vi "MFCDialog.vi"(8 "Error In":errorcluster, 11 "MFC Configuration In":T1={"COM Port"=1, "Timeout (msec)"=100, "Setpoint"=0.0, "Valve State"=enum."Automatic", "Gas"=enum."Air", "Units"=enum."scc/m", "Serial Number"="", "Firmware Version"=""}) -> (0 "Error Out":errorcluster, 2 "Cancelled?":bool, 3 "MFC Configuration Out":T1={"COM Port"=1, "Timeout (msec)"=100, "Setpoint"=0.0, "Valve State"=enum."Automatic", "Gas"=enum."Air", "Units"=enum."scc/m", "Serial Number"="", "Firmware Version"=""})   [LabVIEW 2012]
uses:
  MFCConfiguration.ctl
  libs/Sierra-M100/Public/Controls/ValveState.ctl
  libs/Sierra-M100/Public/Controls/Gas.ctl
  libs/Sierra-M100/Public/Controls/Units.ctl
  libs/LV-Utilities/LV-Utilities.lvlib
  libs/Sierra-M100/Sierra-M100.lvlib
panel:
  in  "COM Port":u8=1
  in  "Valve State":enum16{"Automatic", "Closed", "Purge"}(ring)
  in  "Setpoint":dbl=nan format="%.1f"
  in  "CANCEL":bool
  in  "DONE":bool
  # "COM Port"
  # "Valve State"
  # "Flow Rate"
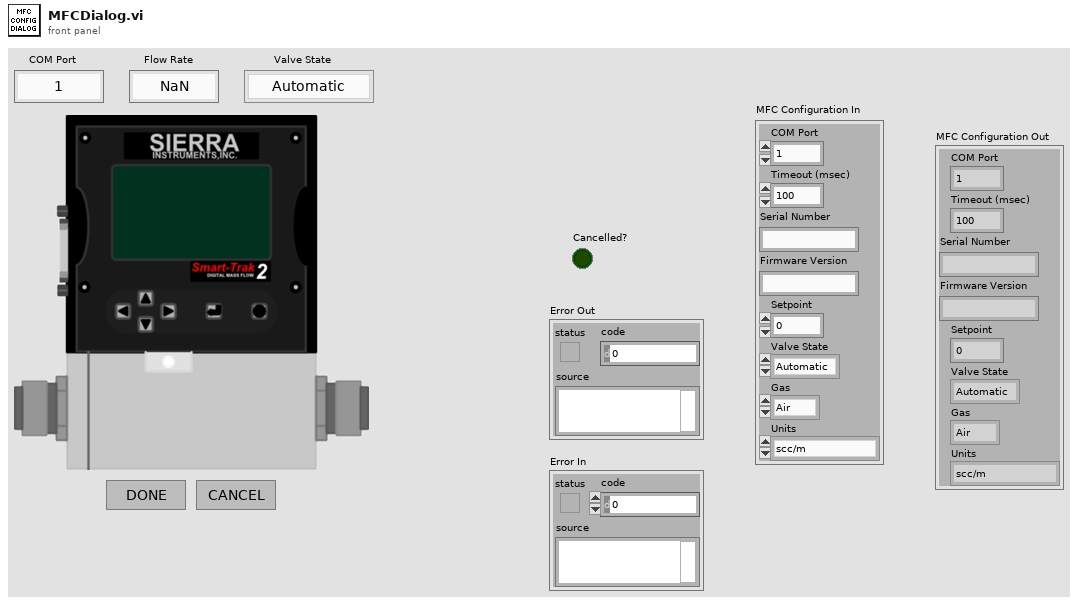
[diagram p1: front panel]
types:
  T1 = typedef "MFCConfiguration.ctl" = cluster{"COM Port":u32, "Timeout (msec)":u32, "Setpoint":dbl, "Valve State":T2, "Gas":T3, "Units":T4, "Serial Number":string, "Firmware Version":string}
  T2 = typedef "Sierra-M100.lvlib/ValveState.ctl" = enum16{"Automatic", "Closed", "Purge"}
  T3 = typedef "Sierra-M100.lvlib/Gas.ctl" = enum16{"Air", "Argon", "CO2", "CO", "Helium", "Hydrogen", "Methane", "Nitrogen", "Nitrous Oxide", "Oxygen"}
  T4 = typedef "Sierra-M100.lvlib/Units.ctl" = enum16{"scc/s", "scc/m", "scc/H", "Ncc/s", "Ncc/m", "Ncc/H", "SCF/s", "SCF/m", "SCF/H", "NM3/s", "NM3/m", "NM3/H", "SM3/s", "SM3/m", "SM3/H", "sl/s", "sl/m", "sl/H", "NL/s", "NL/m", "Nl/H", "g/s", "g/m", "g/H", "kg/s", "kg/m", "kg/H", "lb/s", "lb/m", "lb/H"}
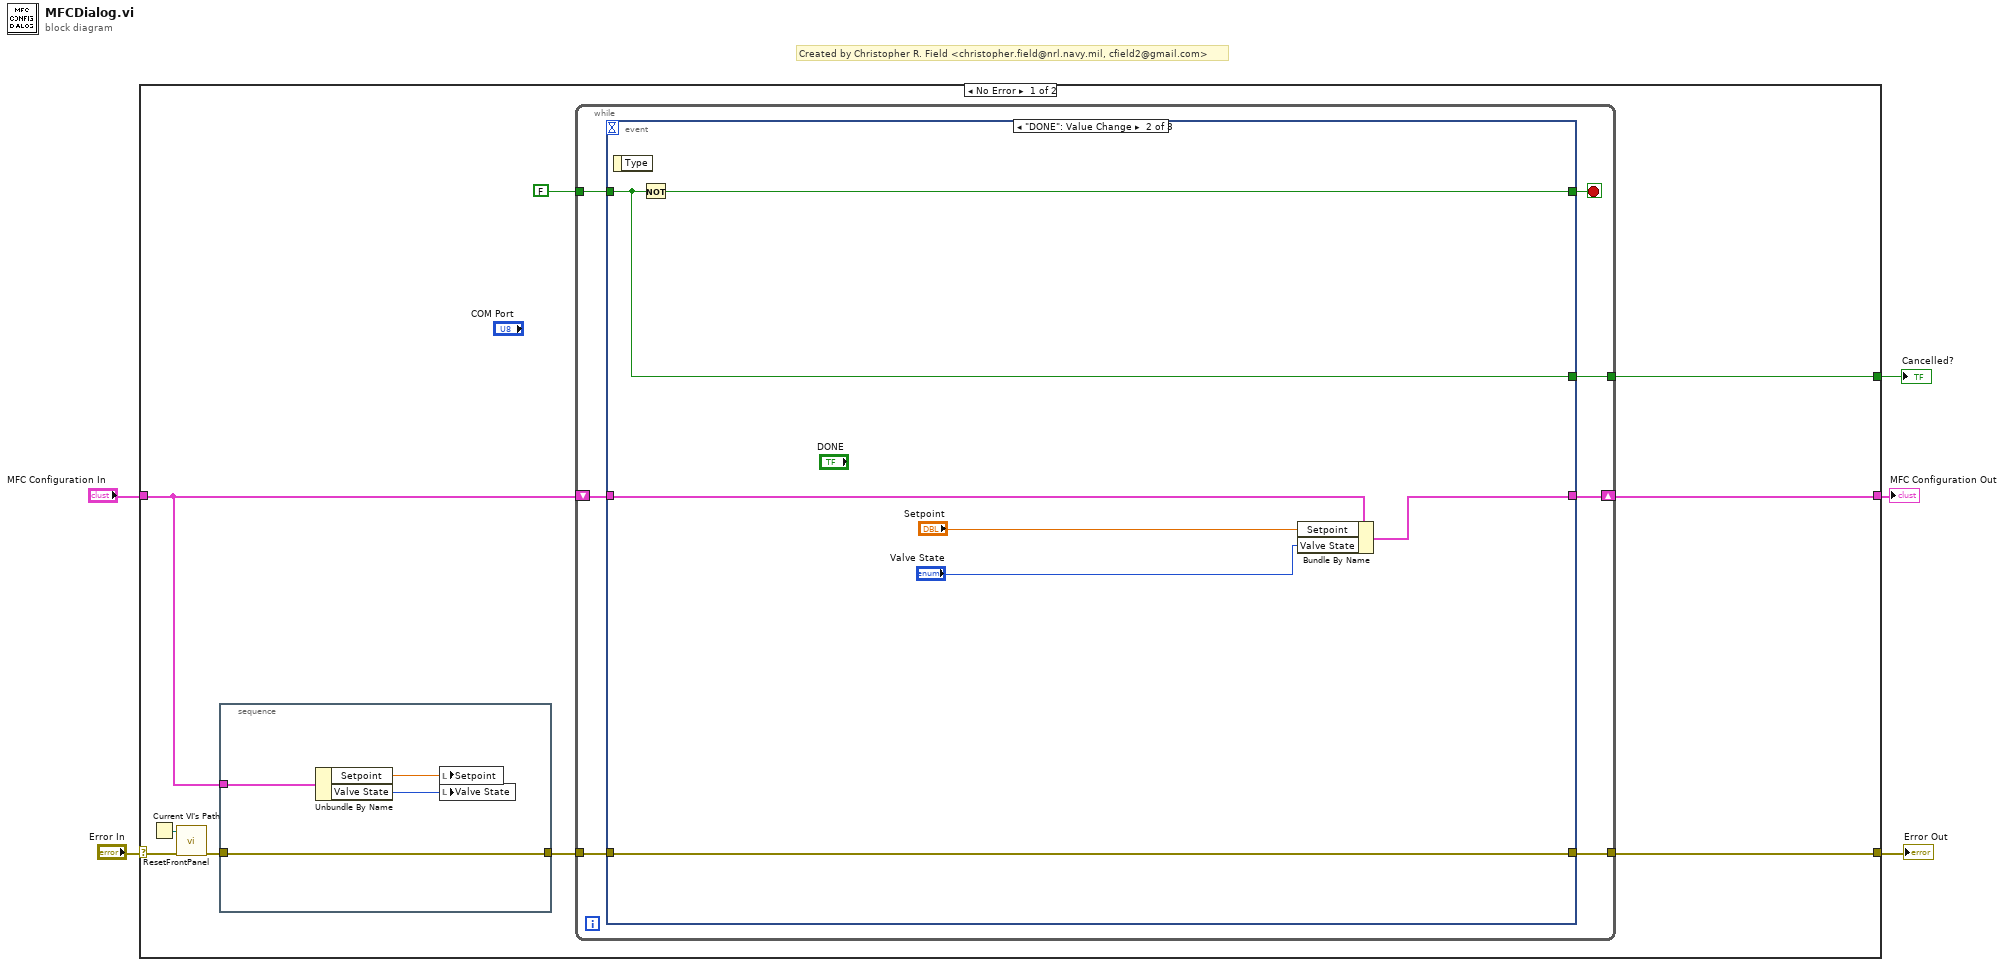
[diagram p0: block diagram]
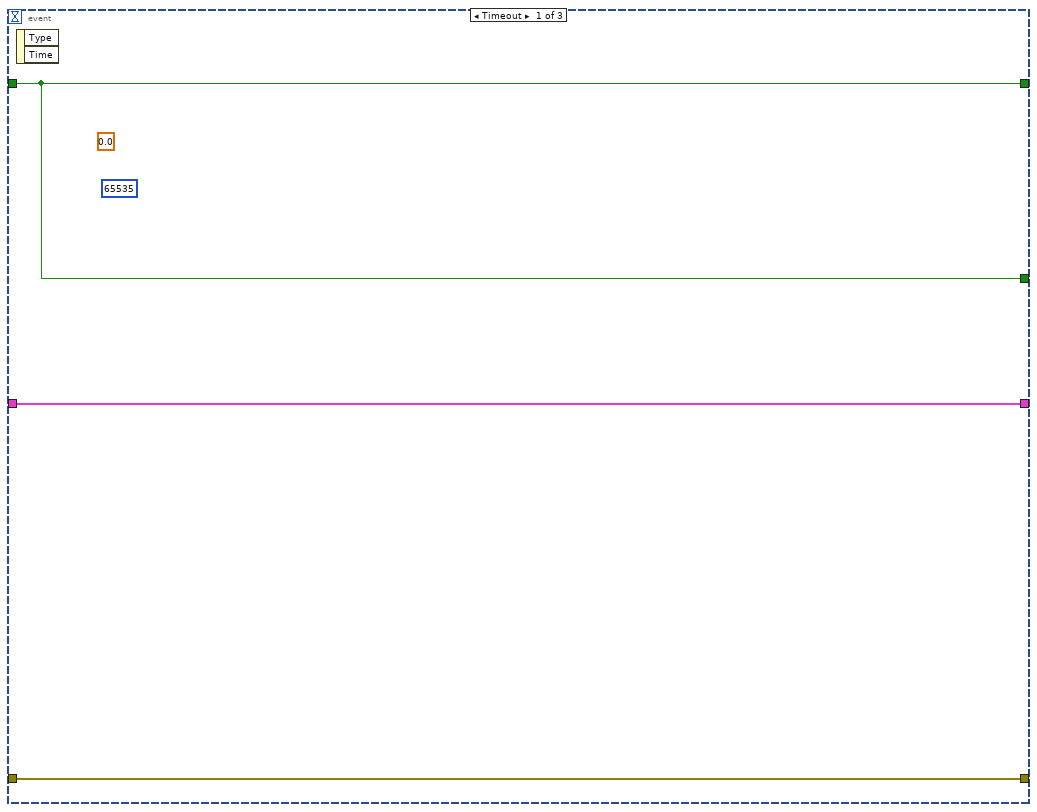
[diagram p2: hidden frame]
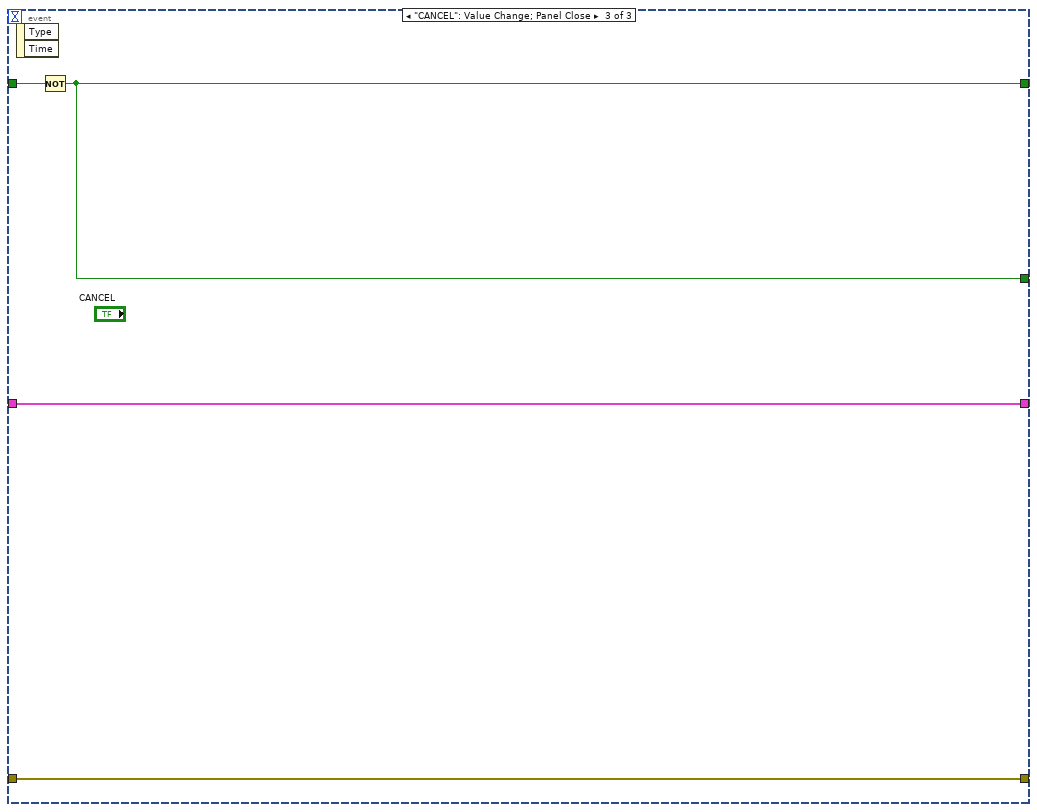
[diagram p3: hidden frame]
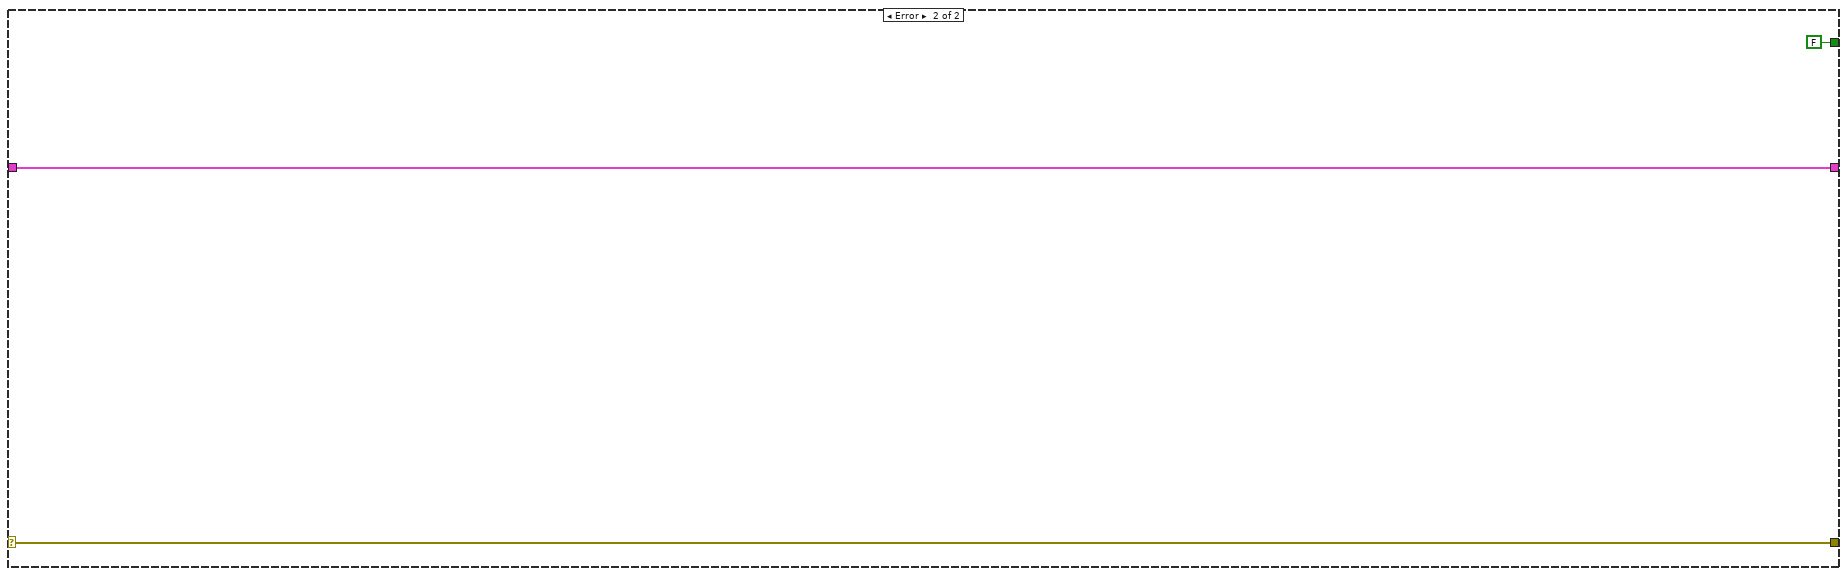
[diagram p4: hidden frame]
diagram:
  # "Created by Christopher R. Field <christopher.field@nrl.navy.mil, cfield2@gmail.com>"
  n1 = case shown="No Error" "Error In" {
    selector: "Error In" -> [w8 w42]
    tunnel: [w11 FALSE] -> w5
    tunnel: [w10 w42] -> w4
    tunnel: "MFC Configuration In" -> [w7 w40]
    tunnel: [w6 w40] -> w1
    frame No Error {
      n2 = Current VI's Path() -> (path=w9:path)
      n3 = call "ResetFrontPanel.vi"("Error In"=w8, "VI Path"=w9) -> ("Error Out"=w13:errorcluster)  [unwired: 9 in]
      n4 = stacked-sequence {
        tunnel: w13 -> [w18]
        tunnel: [w18] -> w12
        tunnel: w7 -> [w17]
        frame #0 {
          n5 = Unbundle By Name(w17) -> ("Setpoint"=w16:dbl, "Valve State"=w15:T2)
          n6 = local write "Setpoint"(w16) -> ()
          n7 = local write "Valve State"(w15) -> ()
        }
      }
      n8 = while {
        tunnel: FALSE -> [w25]
        tunnel: [w23] -> w11
        tunnel: w12 -> [w22]
        tunnel: [w21] -> w10
        shift-right: [w19] -> w6
        shift-left: w7 -> [w20]
        stop <- w24 stop-if-true
        n9 = event shown="[1] \"DONE\": Value Change" {
          selector: _ -> [_ _ _]
          dyn-events: _ -> [_ _ _]
          timeout: _ -> [_ _ _]
          tunnel: w25 -> [w28 w34 w39]
          tunnel: [w28 w35 w38] -> w24
          tunnel: [w28 w34 w38] -> w23
          tunnel: w22 -> [w27 w33 w37]
          tunnel: [w27 w33 w37] -> w21
          tunnel: w20 -> [w26 w29 w36]
          tunnel: [w26 w30 w36] -> w19
          event Timeout {
            (unwired) u16 65535
            (unwired) 0.0 ("Setpoint (mL/min)")
            n10 = event-data() -> ()  [unwired: 1 in, 2 out]
          }
          event "DONE": Value Change {
            n11 = event-data() -> ()  [unwired: 1 in, 1 out]
            n12 = Not(x=w34) -> (.not. x?=w35:bool)
            n13 = Bundle By Name(cluster=w29, "Setpoint"="Setpoint", "Valve State"="Valve State") -> (w30:T1)
          }
          event "CANCEL": Value Change; Panel Close {
            n14 = event-data() -> ()  [unwired: 1 in, 2 out]
            n15 = Not(x=w39) -> (.not. x?=w38:bool)
          }
        }
      }
    }
    frame Error {
    }
  }
  "Cancelled?" <- w5
  "Error Out" <- w4
  "MFC Configuration Out" <- w1
